vi "Ecualizador1.2.vi"() -> ()   [LabVIEW 2020]
uses:
  <vilib>/express/express analysis/Spectral/Block/exnSpectralBlock spectral measurements peak poly.vi
  <vilib>/express/express analysis/Spectral/Block/exnSpectralBlock spectral measurements peak DDT.vi
  <vilib>/express/express analysis/Spectral/XNode/ExpressSpectralMeasurementsBlockNode.xnode
panel:
  in  "stop":bool
  out "Señal de Salida":dynamicdata(graph) caption="Waveform Chart 3"
  out "Señal de Salida Filtrada":dynamicdata(graph)
  out "Waveform Chart":dynamicdata(graph)
  in  "TREBLE":dbl(slide) scale=0.0..10.0
  in  "MIDS":dbl(slide) scale=0.0..10.0
  in  "BASS":dbl(slide) scale=0.0..10.0
  in  "MASTER CONTROL":dbl(slide) scale=0.0..1.0
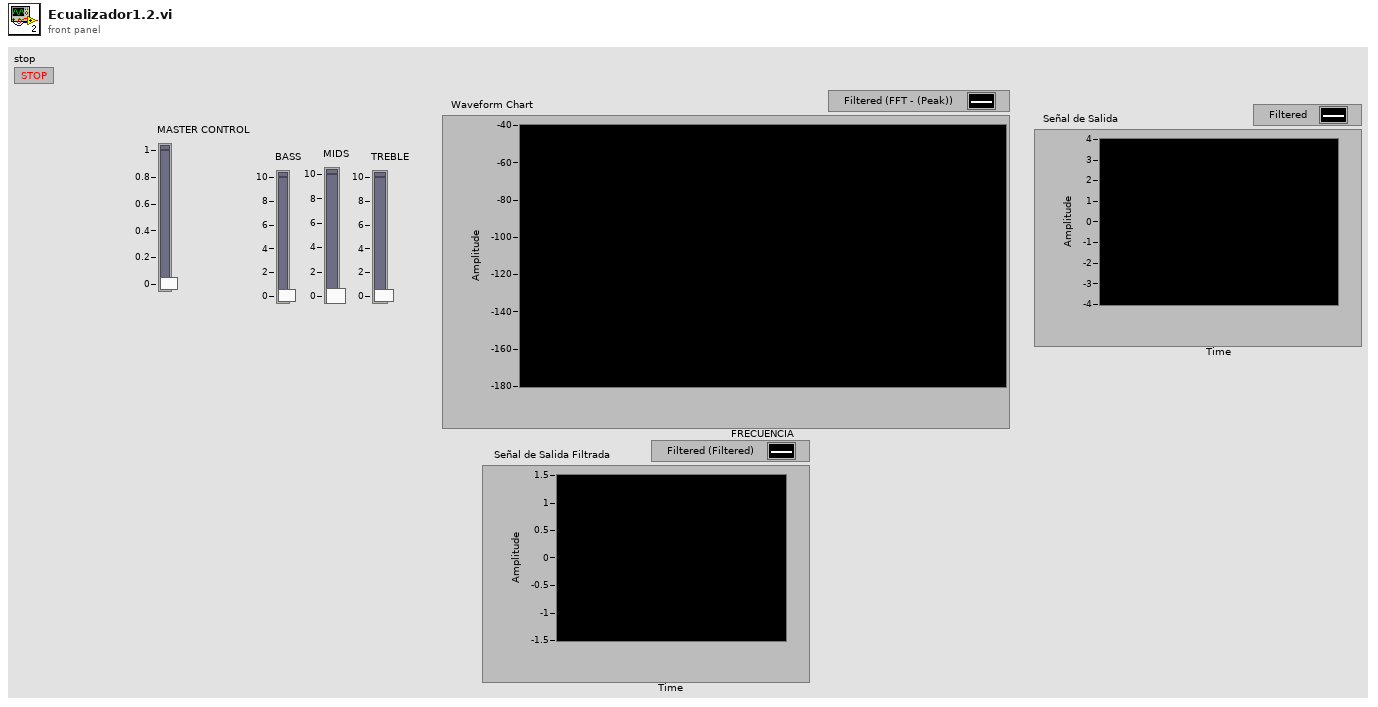
[diagram p1: front panel]
types:
  T1 = cluster{"averaging mode":u16, "weighting mode":u16, "number of averages":u32}
  T2 = cluster{"dB On (F)":bool, "unwrap phase (F)":bool, "convert to degree (F)":bool}
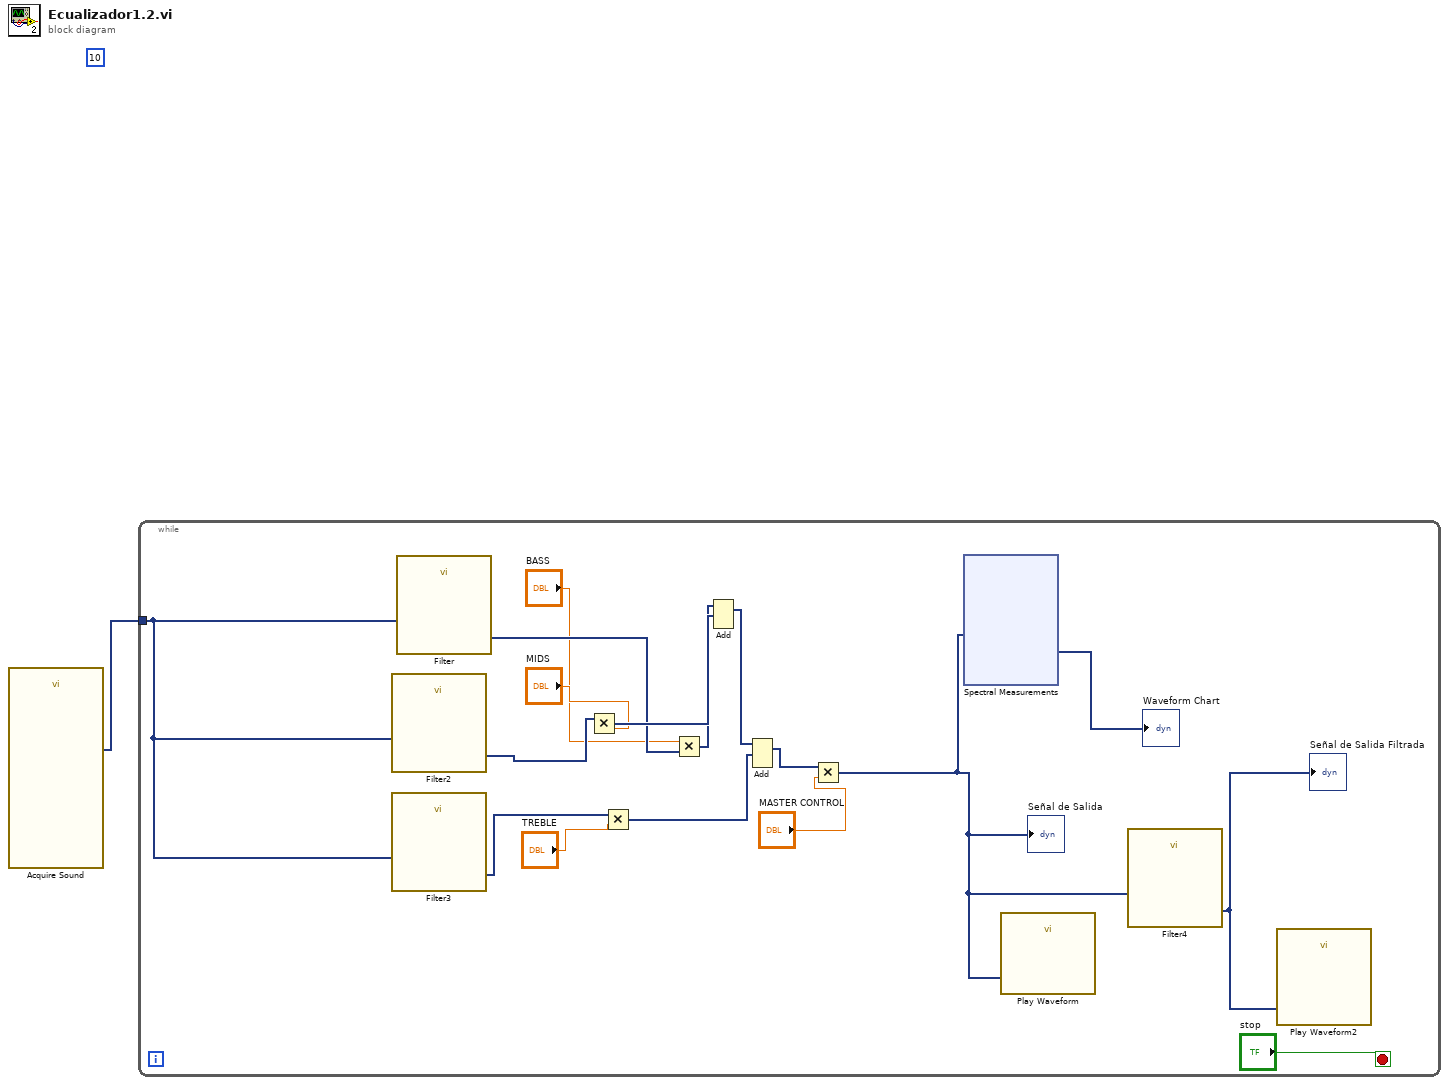
[diagram p0: block diagram]
diagram:
  (unwired) 10
  n1 = call "Acquire Sound"() -> ("Data"=w1:dynamicdata)  [unwired: 18 in, 1 out]
  n2 = while {
    tunnel: w1 -> [w6]
    stop <- "stop" stop-if-true
    n3 = call "Filter2"("Signal"=w6) -> ("Filtered Signal"=w10:dynamicdata)  [unwired: 9 in, 1 out]
    n4 = call "Filter3"("Signal"=w6) -> ("Filtered Signal"=w7:dynamicdata)  [unwired: 9 in, 1 out]
    n5 = call "Filter"("Signal"=w6) -> ("Filtered Signal"=w9:dynamicdata)  [unwired: 9 in, 1 out]
    n6 = Multiply(x=w10, y="MIDS") -> (x*y=w14:dynamicdata)
    n7 = Multiply(x=w7, y="TREBLE") -> (x*y=w16:dynamicdata)
    n8 = Multiply(x="BASS", y=w9) -> (x*y=w13:dynamicdata)
    n9 = Add(1:w14, 2:w13) -> (0:w15:dynamicdata)  [unwired: 1 in, 1 out]
    n10 = Add(1:w16, 2:w15) -> (0:w17:dynamicdata)  [unwired: 1 in, 1 out]
    n11 = Multiply(x=w17, y="MASTER CONTROL") -> (x*y=w2:dynamicdata)
    "Señal de Salida" <- w2
    n12 = xnode "Spectral Measurements"("Signals"=w2) -> ("FFT - (Peak)"=→"Waveform Chart":dynamicdata)  [unwired: 1 in, 2 out]
    n13 = call "Play Waveform"("Data"=w2) -> ()  [unwired: 18 in, 1 out]
    n14 = call "Filter4"("Signal"=w2) -> ("Filtered Signal"=w5:dynamicdata)  [unwired: 9 in, 1 out]
    "Señal de Salida Filtrada" <- w5
    n15 = call "Play Waveform2"("Data"=w5) -> ()  [unwired: 18 in, 1 out]
  }
